vi "Misc-Query Integration-Time.vi"(0 "VISA resource name":refnum<visa-resource-name>, 11 "error in (no error)":errorcluster) -> (3 "medium integration time":dbl format="%^.2e", 4 "VISA resource name out":refnum<visa-resource-name>, 6 "NPLC (medium integration time)":i32, 8 "NPLC (long integration time)":i32, 10 "NPLC (short integration time)":dbl format="%.5f", 13 "short integration time":dbl format="%^.2e", 14 "long integration time":dbl format="%^.2e", 15 "error out":errorcluster)   [LabVIEW 2016, in "Agilent 415X Series.lvlib"]
doc: "This VI queries all the current integration time settings (long, medium, short) and the number of power line cycles for all three integration time modes."
uses:
  Agilent 415X Series.lvlib
panel:
  # "(sec)"
  # "(sec)"
  # "(sec)"
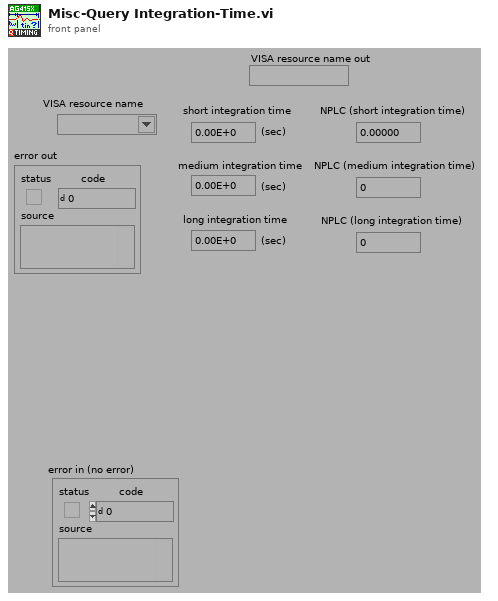
[diagram p1: front panel]
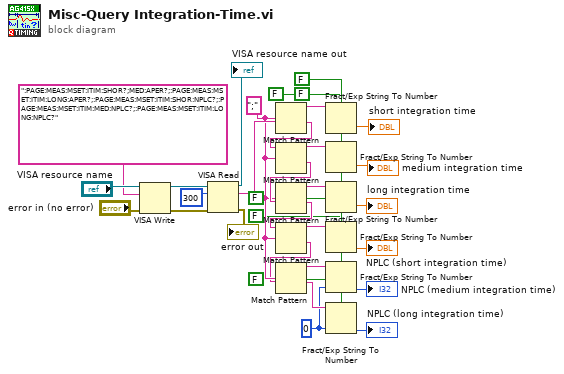
[diagram p0: block diagram]
diagram:
  w8 = 0 ("default (0 U16)")
  w22 = ";"
  n1 = VISA Write(VISA resource name="VISA resource name", write buffer=":PAGE:MEAS:MSET:ITIM:SHOR?;MED:APER?;:PAGE:MEAS:MSET:ITIM:LONG:APER?;:PAGE:MEAS:MSET:ITIM:SHOR:NPLC?;:PAGE:MEAS:MSET:ITIM:MED:NPLC?;:PAGE:MEAS:MSET:ITIM:LONG:NPLC?", error in (no error)="error in (no error)") -> (VISA resource name out=w29:refnum<visa-resource-name>, error out=w30:errorcluster)  [unwired: 1 out]
  n2 = VISA Read(VISA resource name=w29, byte count=300, error in (no error)=w30) -> (VISA resource name out=→"VISA resource name out":refnum<visa-resource-name>, read buffer=w26:string, error out=→"error out":errorcluster)  [unwired: 1 out]
  n3 = Match Pattern(string=w26, regular expression=w22) -> (before substring=w20:string, after substring=w25:string)  [unwired: 1 in, 2 out]
  n4 = Match Pattern(string=w25, regular expression=w22) -> (before substring=w18:string, after substring=w23:string)  [unwired: 1 in, 2 out]
  n5 = Match Pattern(string=w23, regular expression=w22) -> (before substring=w19:string, after substring=w24:string)  [unwired: 1 in, 2 out]
  n6 = Match Pattern(string=w24, regular expression=w22) -> (before substring=w17:string, after substring=w21:string)  [unwired: 1 in, 2 out]
  n7 = Match Pattern(string=w21, regular expression=w22) -> (before substring=w16:string, after substring=w15:string)  [unwired: 1 in, 2 out]
  n8 = Fract/Exp String To Number(use system decimal point (T)=FALSE, string=w20) -> (number=→"short integration time":dbl)  [unwired: 2 in, 1 out]
  n9 = Fract/Exp String To Number(use system decimal point (T)=FALSE, string=w18) -> (number=→"medium integration time":dbl)  [unwired: 2 in, 1 out]
  n10 = Fract/Exp String To Number(use system decimal point (T)=FALSE, string=w19) -> (number=→"long integration time":dbl)  [unwired: 2 in, 1 out]
  n11 = Fract/Exp String To Number(use system decimal point (T)=FALSE, string=w17) -> (number=→"NPLC (short integration time)":dbl)  [unwired: 2 in, 1 out]
  n12 = Fract/Exp String To Number(use system decimal point (T)=FALSE, string=w16, default (0 dbl)=w8) -> (number=→"NPLC (medium integration time)":i32)  [unwired: 1 in, 1 out]
  n13 = Fract/Exp String To Number(use system decimal point (T)=FALSE, string=w15, default (0 dbl)=w8) -> (number=→"NPLC (long integration time)":i32)  [unwired: 1 in, 1 out]
